vi "shif_register.vi"() -> ()   [LabVIEW 2017]
panel:
  out "output array":i32[](array[numeric])
  in  "ms":dbl
  out "ii":dbl
  in  "For loop":dbl
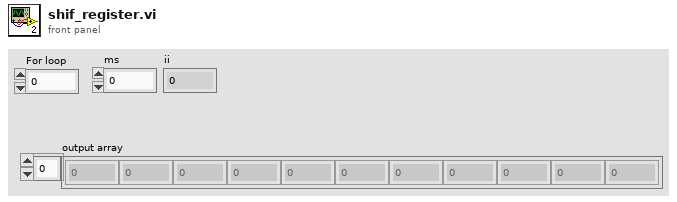
[diagram p1: front panel]
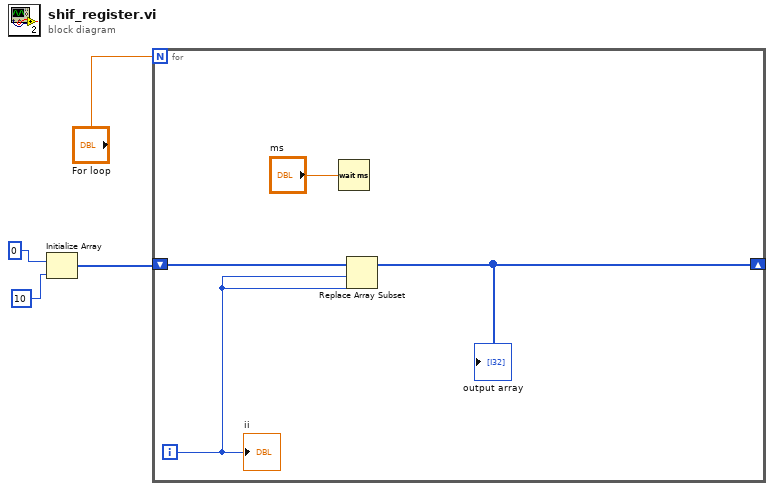
[diagram p0: block diagram]
diagram:
  n1 = Initialize Array(0, 10) -> (w1:i32[])
  n2 = for {
    N: "For loop" -> [_]
    shift-right: [w6] -> _
    shift-left: w1 -> [w7]
    i -> [w5]
    n3 = Wait (ms)(milliseconds to wait="ms") -> ()  [unwired: 1 out]
    n4 = Replace Array Subset(array=w7, new element=w5, index=w5) -> (w6:i32[])
    "output array" <- w6
    "ii" <- w5
  }
